vi "RW utf-8.vi"(1 "Original":string) -> (0 "Decoded":string)   [LabVIEW 2018, in "qingshan.lvlib"]
panel:
  out "utf-8 Encoded":string
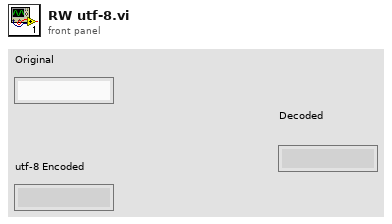
[diagram p1: front panel]
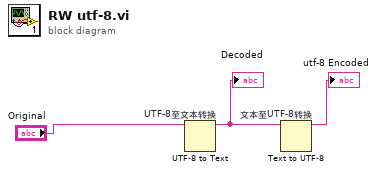
[diagram p0: block diagram]
diagram:
  n1 = UTF-8 to Text "UTF-8至文本转换"(11:"Original") -> (3:w3:string)  [unwired: 2 in, 1 out]
  "Decoded" <- w3
  n2 = Text to UTF-8 "文本至UTF-8转换"(11:w3) -> (3:→"utf-8 Encoded":string)  [unwired: 2 in, 1 out]
